vi "SetPath.vi"(10 "path to VI that identifies classes":path, 11 "GettingStartedWindow.lvlib:Error.lvclass":refnum<class "Error.lvclass">) -> (3 "GettingStartedWindow.lvlib:Error.lvclass 2":refnum<class "Error.lvclass">)   [LabVIEW 2009, in "NavScreen.lvlib" / "Error.lvclass"]
uses:
  Error.lvclass
  Error.lvclass/Error.ctl
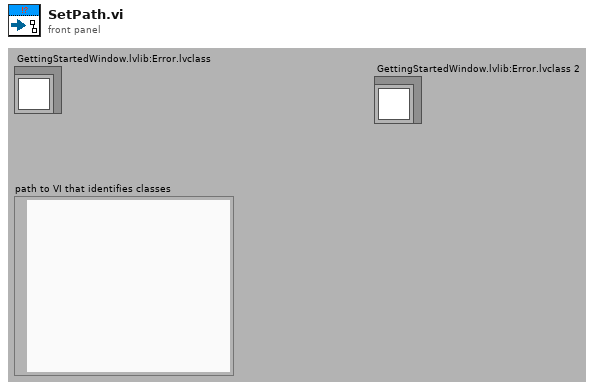
[diagram p1: front panel]
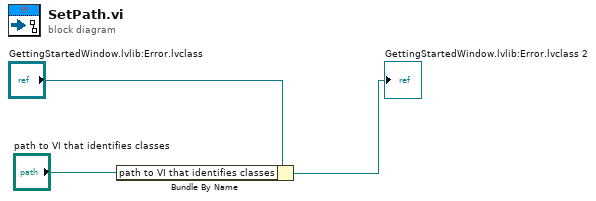
[diagram p0: block diagram]
diagram:
  n1 = Bundle By Name(cluster="GettingStartedWindow.lvlib:Error.lvclass", "path to VI that identifies classes"="path to VI that identifies classes") -> (→"GettingStartedWindow.lvlib:Error.lvclass 2":refnum<class "Error.lvclass">)
